vi "Static Timer Reference.vi"() -> (4 "Branched Timer Index":T1)   [LabVIEW 2010, in "timerExts.lvlib"]
uses:
  timerExts.lvlib
  Branched Timer.ctl
  CLIB/CRef/CRef.lvlib
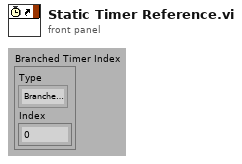
[diagram p1: front panel]
types:
  T1 = typedef "timerExts.lvlib/Branched Timer.ctl" = cluster{"Type":enum8{"Branched Timer", "NXT Timer"}, "Index":u16}
  T2 = typedef "CRef.lvlib/U32 CReference.ctl" = cluster{"Generic CRef Address":u16, "Type":enum8{"Null", "Boolean", "U8", "I8", "U16", "I16", "U32", "I32", "U64", "I64", "Single", "Double", "Extended", "CSG", "CDB", "CXT", "Invalid Def", "U8(Def)", "I8(Def)", "U16(Def)", "I16(Def)", "U32(Def)"}}
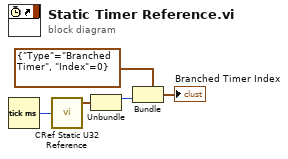
[diagram p0: block diagram]
diagram:
  n1 = Tick Count (ms)() -> (millisecond timer value=w3:u32)
  n2 = call "CRef Static U32 Reference.vi"("Initial Value (0)"=w3) -> ("U32 CReference"=w2:T2)  [unwired: 4 in]
  n3 = Unbundle(w2) -> ("Generic CRef Address"=w1:u16)  [unwired: 1 out]
  n4 = Bundle(cluster=T1 {"Type"=enum."Branched Timer", "Index"=0} ("Branched Timer Index 2"), "Index"=w1) -> (→"Branched Timer Index":T1)  [unwired: 1 in]
